vi "TEST - Set Cluster Element by Name.vi"(8 "error in (no error)":errorcluster) -> (0 "error out":errorcluster, 2 "pass":bool)   [LabVIEW 2020]
panel:
  out "Failures":T1(array[cluster])
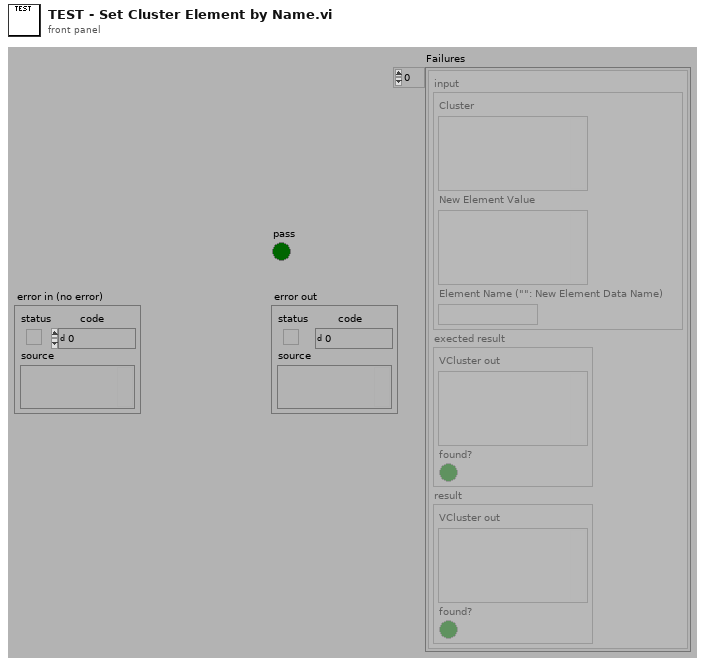
[diagram p1: front panel]
types:
  T1 = cluster{"input":cluster{"Cluster":variant, "New Element Value":variant, "Element Name (\"\": New Element Data Name)":string}, "exected result":cluster{"VCluster out":variant, "found?":bool}, "result":cluster{"VCluster out":variant, "found?":bool}}[]
  T2 = cluster{"input":cluster{"Cluster":variant, "New Element Value":variant, "Element Name (\"\": New Element Data Name)":string}, "exected result":cluster{"VCluster out":variant, "found?":bool}, "result":cluster{"VCluster out":variant, "found?":bool}}
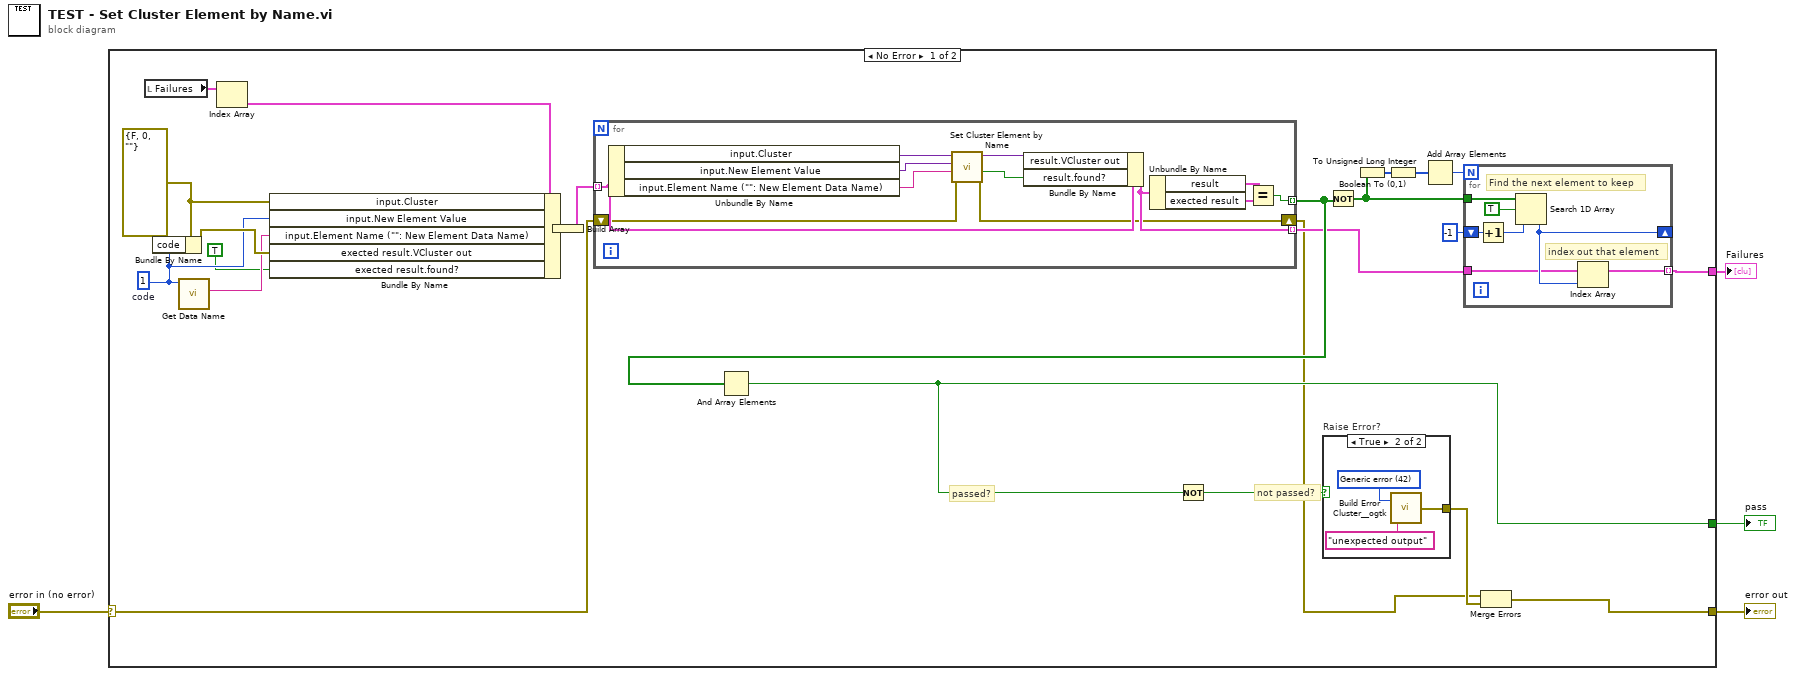
[diagram p0: block diagram]
diagram:
  n1 = case shown="No Error" "error in (no error)" {
    selector: "error in (no error)" -> [w13 w50]
    tunnel: [w24 _] -> w4
    tunnel: [w27 w50] -> w2
    tunnel: [w16 _] -> w1
    frame No Error {
      w9 = errorcluster {"status"=FALSE, "code"=0, "source"=""} ("error in (no error)")
      w7 = 1  # code
      # "not passed?"
      # "passed?"
      n2 = local read "Failures"() -> (w11:T1)
      n3 = Bundle By Name(cluster=w9, "code"=w7) -> (w8:errorcluster)
      n4 = call "Get Data Name.vi"("Data"=w7) -> ("Data Name"=w6:string)  [unwired: 8 in, 2 out]
      n5 = Index Array(array=w11) -> (element=w10:T2)  [unwired: 1 in]
      n6 = Bundle By Name(cluster=w10, "input.Cluster"=w9, "input.New Element Value"=w7, "input.Element Name (\"\": New Element Data Name)"=w6, "exected result.VCluster out"=w8, "exected result.found?"=TRUE) -> (w15:T2)
      n7 = Build Array(w15) -> (w14:T1)
      n8 = for {
        tunnel: w14 -> [w45] mode=indexing
        tunnel: [w46] -> w18 mode=indexing
        tunnel: [w44] -> w17 mode=indexing
        shift-right: [w40] -> w12
        shift-left: w13 -> [w41]
        n9 = Unbundle By Name(w45) -> ("input.Cluster"=w39:variant, "input.New Element Value"=w38:variant, "input.Element Name (\"\": New Element Data Name)"=w37:string)
        n10 = call "Set Cluster Element by Name.vi"("error in (no error)"=w41, "Element Name (\"\": New Element Data Name)"=w37, "New Element Value"=w38, "Cluster"=w39) -> ("error out"=w40:errorcluster, "found?"=w36:bool, "VCluster out"=w35:variant)  [unwired: 5 in]
        n11 = Bundle By Name(cluster=w45, "result.VCluster out"=w35, "result.found?"=w36) -> (w44:T2)
        n12 = Unbundle By Name(w44) -> ("result"=w43:cluster{"VCluster out":variant, "found?":bool}, "exected result"=w42:cluster{"VCluster out":variant, "found?":bool})
        n13 = Equal?(x=w43, y=w42) -> (x = y?=w46:bool)
      }
      n14 = And Array Elements(Boolean array=w18) -> (logical AND=w24:bool)
      n15 = Not(x=w24) -> (.not. x?=w25:bool)
      n16 = case "Raise Error?" shown="True" w25 {
        tunnel: [_ w47] -> w26
        frame False {
        }
        frame True {
          w48 = 42 items=["No error", "Argument error", "Memory is full", "Out of zone", "End of file", "File already open", "Generic file I/O error", "File not found", "File permission error", "Disk is full", "Duplicate path", "Too many files open", "System feature not enabled", "Resource file not found", "Cannot add resource", "Resource not found", "Image not found", "Image memory error", "Pen does not exist", "Config type invalid", "Config token not found", "Config parse error", "Config memory error", "Bad external code format", "Bad external code offset", "External code not present", "Null window", "Destroy window error", "Null menu", "Print aborted", "Bad print record", "Print driver error", "Windows error during printing", "Memory error during printing", "Print dialog error", "Generic print error", "Invalid device refnum", "Device not found", "Device parameter error", "Device unit error", "Cannot open device", "Device call aborted", "Generic error", "Cancelled by user", "Object ID too low", "Object ID too high", "Object not in heap", "Unknown heap", "Unknown object (invalid DefProc)", "Unknown object (DefProc not in table)", "Message out of range", "Invalid (null) method", "Unknown message", "Manager call not supported", "Bad address", "Network operation in progress", "Network operation timed out", "Connection is busy", "Network attribute not supported", "Network error", "Address in use", "System out of memory", "Connection aborted", "Connection refused", "Not connected", "Already connected", "Connection closed", "Initialization error (interapplication manager)", "Bad occurrence", "Wait on unbound occurrence handler", "Occurrence queue overflow", "Datalog type conflict", "Unused", "Unrecognized type (interapplication manager)", "Memory corrupt", "Failed to make temporary DLL", "Old CIN version", "Drag socket not found", "Failed to load drop-object", "Failed to register OLE object", "Failed to release OLE object", "Format specifier type mismatch", "Unknown format specifier", "Too few format specifiers", "Too many format specifiers", "Scan failed", "Newer CIN version", "Error converting to variant", "Runtime menu error", "Password tampered", "Variant attribute not found", "Incompatible variant data type", "Event data is not available", "Event Store is not present", "Occurrence is not found", "Event Queue is not created", "Event info is not available", "Refnum passed is NULL", "Error retrieving Class GUID", "Error retrieving CoClass GUID", "Error retrieving TypeLib GUID.", "Bad built application magic bytes.", "Specific driver is different from the specific driver associated with the Logical Name.", "There is no session opened to the class driver.", "Max Error", "MAX - Error with config objects", "MAX - Error loading configuration", "MAX - Group not supported"]
          n17 = call <userlib>:"Build Error Cluster__ogtk.vi"("String to Prepend to source (\"\")"="unexpected output" ("String to Prepend to source (\"\")"), "code"=w48) -> ("error out"=w47:errorcluster)
        }
      }
      n18 = Not(x=w18) -> (.not. x?=w20:bool[])
      n19 = Boolean To (0,1)(Boolean=w20) -> (0, 1=w21:i16[])
      n20 = To Unsigned Long Integer(number=w21) -> (unsigned 32bit integer=w19:u32[])
      n21 = Add Array Elements(numeric array=w19) -> (sum=w22:u32)
      n22 = for {
        N: w22 -> [_]
        tunnel: w17 -> [w30]
        tunnel: w20 -> [w34]
        shift-right: [w31] -> _
        shift-left: -1 ("start index (0)") -> [w32]
        tunnel: [w29] -> w16 mode=indexing
        # "index out that element"
        # "Find the next element to keep"
        n23 = Increment(x=w32) -> (x+1=w28:i32)
        n24 = Search 1D Array(1D array=w34, element=TRUE, start index (0)=w28) -> (index of element=w31:i32)
        n25 = Index Array(array=w30, index=w31) -> (element=w29:T2)
      }
      n26 = Merge Errors(w12, w26) -> (w27:errorcluster)
    }
    frame Error {
    }
  }
  "pass" <- w4
  "error out" <- w2
  "Failures" <- w1
